vi "ADD DFS Items All.vi"(11 "Tree in":refnum<class "Tree.lvclass">) -> (3 "Tree out":refnum<class "Tree.lvclass">)   [LabVIEW 2019, in "Tree.lvclass"]
uses:
  Tree.lvclass
  Type Def/Tree Item.ctl
  Tree.lvclass/Tree.ctl
  Type Def/LV Original TreeItem.ctl
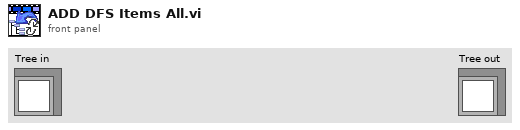
[diagram p1: front panel]
types:
  T1 = typedef "Tree Item.ctl" = cluster{"Parent Tag":string, "Tag":string, "Left Cell":string, "Cells Text":string[], "BFS Index":i32[], "Graph Index":i32, "Item Indent":i32}
  T2 = typedef "LV Original TreeItem.ctl" = cluster{"Left Cell String":string, "Child Text":string[], "Child Tag":string, "Item Indent":i32, "Child Only?":bool, "Glyph Index":i32}
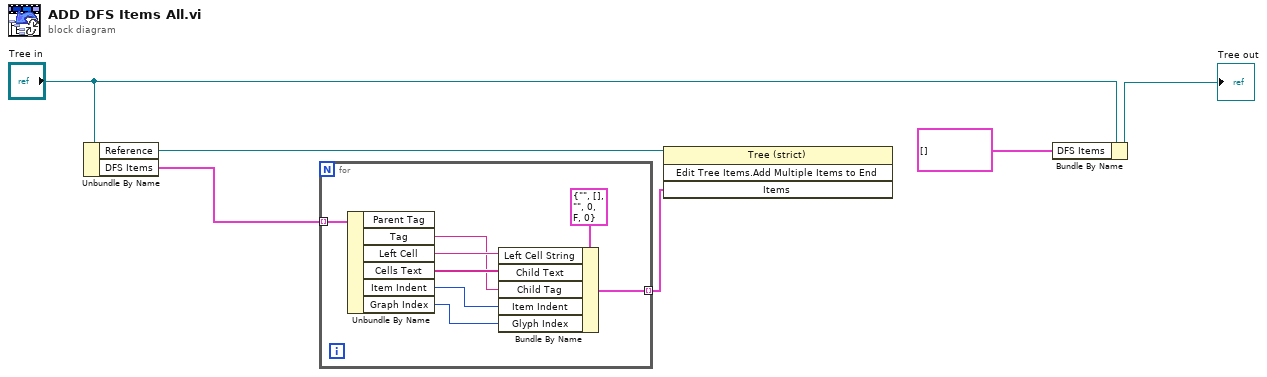
[diagram p0: block diagram]
diagram:
  n1 = Unbundle By Name("Tree in") -> ("Reference"=w6:refnum<vi>, "DFS Items"=w5:T1[])
  n2 = for {
    tunnel: w5 -> [w14] mode=indexing
    tunnel: [w8] -> w1 mode=indexing
    n3 = Unbundle By Name(w14) -> ("Tag"=w11:string, "Left Cell"=w13:string, "Cells Text"=w12:string[], "Item Indent"=w10:i32, "Graph Index"=w9:i32)  [unwired: 1 out]
    n4 = Bundle By Name(cluster=T2 {"Left Cell String"="", "Child Text"=[], "Child Tag"="", "Item Indent"=0, "Child Only?"=FALSE, "Glyph Index"=0} ("Item"), "Left Cell String"=w13, "Child Text"=w12, "Child Tag"=w11, "Item Indent"=w10, "Glyph Index"=w9) -> (w8:T2)
  }
  n5 = invoke class="Tree (strict)" method="Edit Tree Items.Add Multiple Items to End"(reference=w6, "Items"=w1) -> ()  [unwired: 2 in, 4 out]
  n6 = Bundle By Name(cluster="Tree in", "DFS Items"=T1[] [] ("Multi Items")) -> (→"Tree out":refnum<class "Tree.lvclass">)
